vi "LakeShore 370 Curve Manager.vi"(11 "VISA session":refnum<visa-resource-name>) -> ()   [LabVIEW 2020]
doc: "VI to manage calibration curves in Lakeshore model 370 AC resistance Bridge. It will upload, download and display or delete curves. It will always delete a curve before uploading so the input setup may have to be reset after an upload.\nScott Hannahs, <sth@magnet.fsu.edu> NHMFL-FSU, May 2003"
uses:
  Misc Extras/Manufacturer Drivers/LakeShore/Lake Shore Cryotronics 336/Public/Utility/Data Format.ctl
  Sub Controls/ThermListIndex.ctl
  Misc Extras/Manufacturer Drivers/LakeShore/Lake Shore Cryotronics 370/Lake Shore Cryotronics 370.lvlib
panel:
  in  "Done2":bool
  out "XY Graph":cluster{dbl[], dbl[]}(graph)
  out "Curve #":i32[](array[numeric])
  in  "ThermListIndex":T1 max=40 step=20
  in  "stop":bool
  in  "Replace":bool[](array[boolean])=[FALSE, FALSE, FALSE, FALSE, FALSE, FALSE, FALSE, FALSE, FALSE, FALSE, FALSE, FALSE, FALSE, FALSE, FALSE, FALSE, FALSE, FALSE, FALSE, FALSE]
  in  "View":bool[](array[boolean])=[FALSE, FALSE, FALSE, FALSE, FALSE, FALSE, FALSE, FALSE, FALSE, FALSE, FALSE, FALSE, FALSE, FALSE, FALSE, FALSE, FALSE, FALSE, FALSE, FALSE]
  in  "Delete":bool[](array[boolean])=[FALSE, FALSE, FALSE, FALSE, FALSE, FALSE, FALSE, FALSE, FALSE, FALSE, FALSE, FALSE, FALSE, FALSE, FALSE, FALSE, FALSE, FALSE, FALSE, FALSE]
  out "Thermometer List":T3(array[cluster]) {"Temp. Coef" items=["????", "Negative", "Positive"]; "Setpoint Limit" format="%.4f"; "Data Format" items=["mV/K"=1, "V/K"=2, "Ω/K"=3, "Log Ω/K"=4]}
  out "Model":string="LakeShore Model 370"
  out "Info":string="S/N #000000, Software Date: 20030622"
  # "Name"
  # "Serial #"
  # "Data Format"
  # "Setpoint Limit"
  # "Temp. Coef"
  # "`"
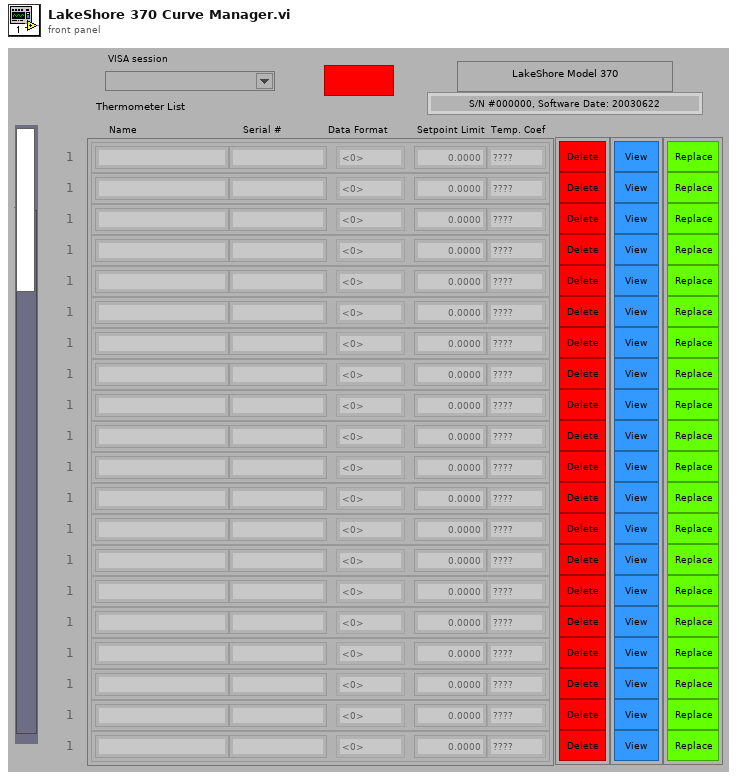
[diagram p1: front panel]
types:
  T1 = typedef "ThermListIndex.ctl" = u32
  T2 = typedef "Data Format.ctl" = u16
  T3 = cluster{"Name":string, "Serial #":string, "Data Format":T2, "Setpoint Limit":dbl, "Temp. Coef":u16}[]
  T4 = cluster{"Curve ID":string, "Serial Number":string, "Data Format":T2, "Setpoint Limit":dbl, "Temp. Coef":u16}[]
  T5 = enum8{"Enabled", "Disabled", "Disabled and Grayed Out"}
  T6 = cluster{"Curve ID":string, "Serial Number":string, "Data Format":T2, "Setpoint Limit":dbl, "Temp. Coef":u16}
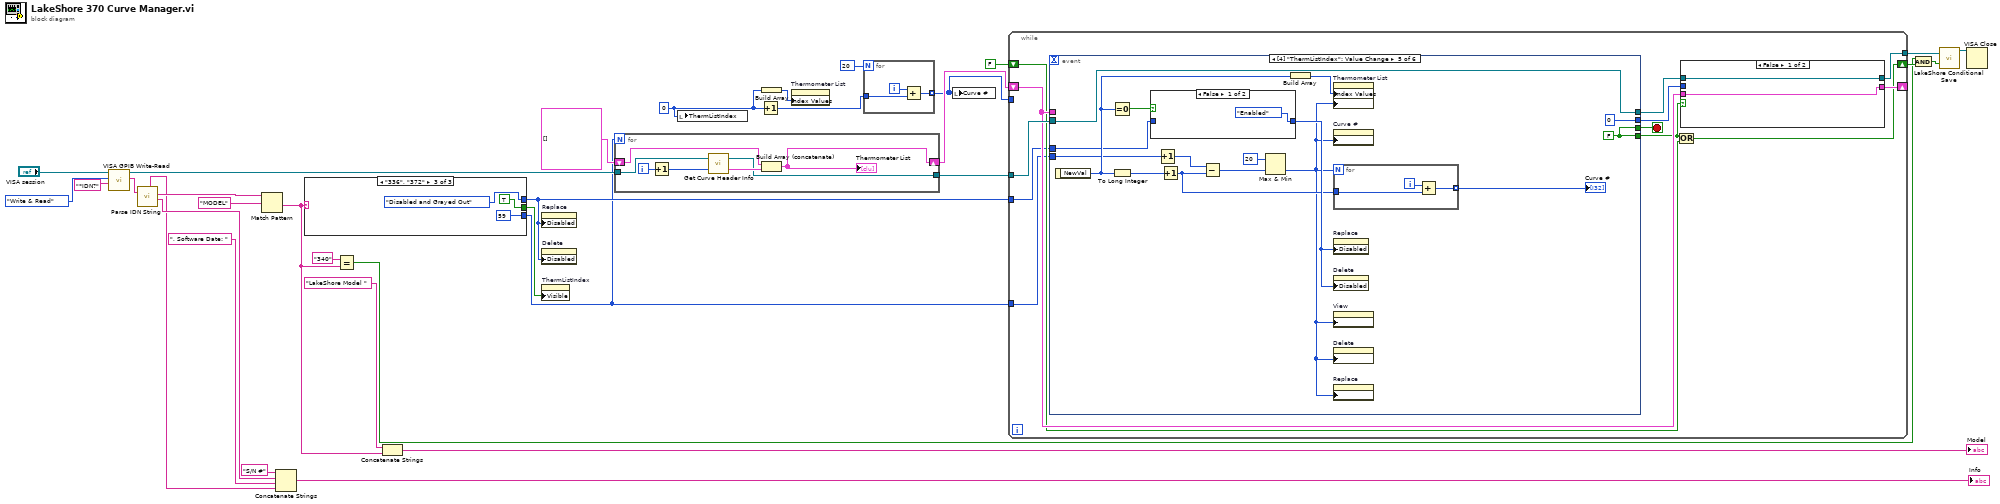
[diagram p0: block diagram]
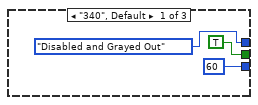
[diagram p2: hidden frame]
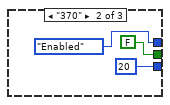
[diagram p3: hidden frame]
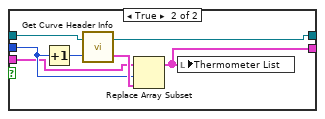
[diagram p4: hidden frame]
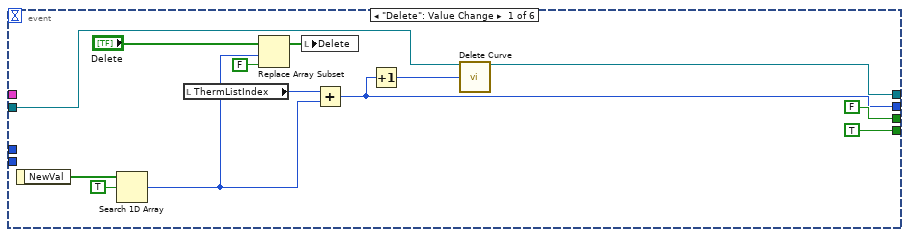
[diagram p5: hidden frame]
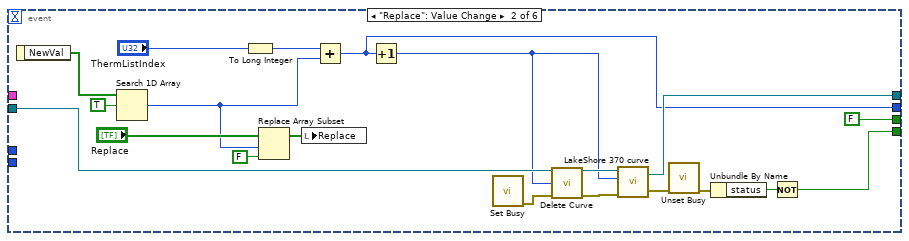
[diagram p6: hidden frame]
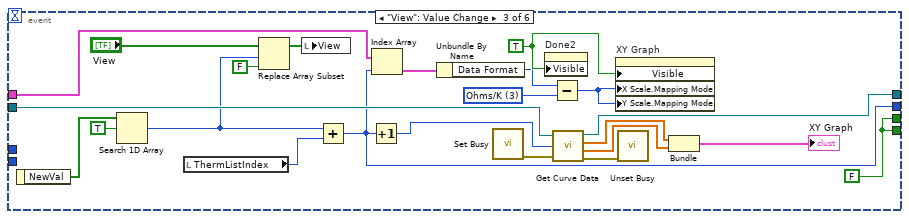
[diagram p7: hidden frame]
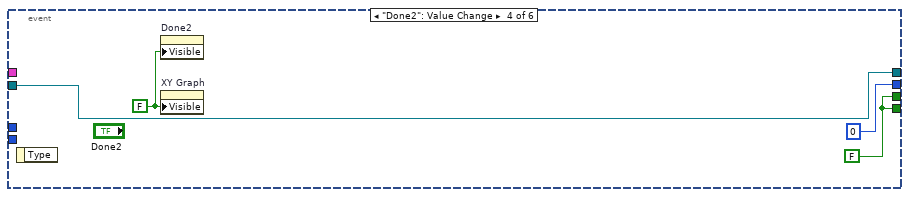
[diagram p8: hidden frame]
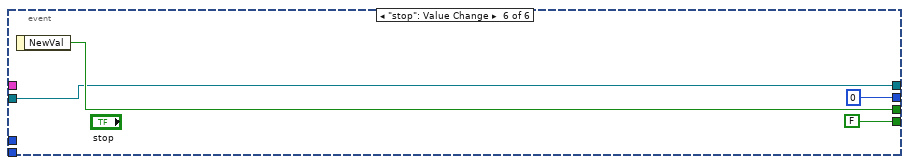
[diagram p10: hidden frame]
diagram:
  w22 = u32 0
  n1 = call "VISA GPIB Write-Read.vi"("Command"="*IDN?" ("String to Write"), "Action"=enum16{"Write", "Read", "Write & Read"}."Write & Read", "VISA resource name"="VISA session") -> ("String Returned"=w10:string, "dup VISA Session"=w27:refnum<visa-resource-name>)  [unwired: 5 in, 2 out]
  n2 = call "Parse IDN String.vi"("IDN String"=w10) -> ("Info"=w7:string, "Model"=w9:string, "Revision"=w6:string)  [unwired: 1 in, 2 out]
  n3 = Match Pattern(string=w9, regular expression="MODEL" ("search string")) -> (after substring=w4:string)  [unwired: 1 in, 3 out]
  n4 = Concatenate Strings("S/N #" ("string"), w7, ", Software Date: " ("string"), w6) -> (→"Info":string)
  n5 = case shown="\"336\", \"372\"" w4 {
    tunnel: [60 20 59] -> w1
    tunnel: [TRUE ("Visible") FALSE ("Visible") TRUE ("Visible")] -> w3
    tunnel: [T5."Disabled and Grayed Out" ("Disabled") T5."Enabled" ("Disabled") T5."Disabled and Grayed Out" ("Disabled")] -> w2
    frame "340", Default {
    }
    frame "370" {
    }
    frame "336", "372" {
    }
  }
  n6 = Equal?(x="340" ("regular expression"), y=w4) -> (x = y?=w13:bool)
  n7 = Concatenate Strings("LakeShore Model " ("string"), w4) -> (→"Model":string)
  n8 = property on="Replace" class="Arr"("Disabled"=w2) -> ()  [unwired: 2 in, 2 out]
  n9 = property on="Delete" class="Arr"("Disabled"=w2) -> ()  [unwired: 2 in, 2 out]
  n10 = property on="ThermListIndex" class="Slide (strict)"("Visible"=w3) -> ()  [unwired: 2 in, 2 out]
  n11 = for {
    N: w1 -> [_]
    tunnel: w27 -> [w49]
    shift-right: [w44] -> w32
    shift-left: T4 [] -> [w43]
    tunnel: [w45] -> w33
    i -> [w48]
    n12 = Increment(x=w48) -> (x+1=w47:i32)
    n13 = call "Get Curve Header Info.vi"("Curve #"=w47, "VISA session"=w49) -> ("Cluster"=w46:T6, "dup VISA session"=w45:refnum<visa-resource-name>)
    n14 = Build Array (concatenate)(w43, w46) -> (w44:T4)
    "Thermometer List" <- w44
  }
  n15 = local write "ThermListIndex"(w22) -> ()
  n16 = Increment(x=w22) -> (x+1=w25:u32)
  n17 = Build Array(w22) -> (w24:u32[])
  n18 = property on="Thermometer List" class="Arr (strict)"("Index Values"=w24) -> ()  [unwired: 2 in, 2 out]
  n19 = for {
    N: 20 -> [_]
    tunnel: w25 -> [w52]
    tunnel: [w50] -> w23 mode=indexing
    i -> [w51]
    n20 = Add(x=w51, y=w52) -> (x+y=w50:u32)
  }
  n21 = local write "Curve #"(w23) -> ()
  n22 = while {
    tunnel: w33 -> [w64]
    shift-right: [w59] -> _
    shift-left: w32 -> [w60]
    tunnel: [w58] -> w18
    tunnel: w23 -> [_]
    shift-right: [w57] -> w20
    shift-left: FALSE ("NewVal") -> [w55]
    tunnel: w2 -> [w54]
    tunnel: w1 -> [w53]
    stop <- w61 stop-if-true
    n23 = event shown="[4] \"ThermListIndex\": Value Change" {
      selector: _ -> [_ _ _ _ _ _]
      dyn-events: _ -> [_ _ _ _ _ _]
      timeout: _ -> [_ _ _ _ _ _]
      tunnel: w64 -> [w84 w90 w127 w130 w149 w156]
      tunnel: [TRUE ("NewVal") w92 w124 w132 w147 FALSE] -> w56
      tunnel: [w74 w97 w109 0 ("index of element") 0 ("index of element") 0 ("index of element")] -> w63
      tunnel: [w83 w104 w126 w130 w149 w156] -> w62
      tunnel: [FALSE ("NewVal") FALSE ("NewVal") w124 w132 w147 w158] -> w61
      tunnel: w60 -> [_ _ w125 _ _ _]
      tunnel: w54 -> [_ _ _ _ w142 _]
      tunnel: w53 -> [_ _ _ _ w138 _]
      event "Delete": Value Change {
        n24 = event-data() -> ("NewVal"=w86:bool[])  [unwired: 1 in]
        n25 = Search 1D Array(1D array=w86, element=TRUE) -> (index of element=w75:i32)  [unwired: 1 in]
        n26 = local read "ThermListIndex"() -> (w76:T1)
        n27 = Replace Array Subset(array="Delete", new element=FALSE ("new element/subarray"), index=w75) -> (w78:bool[])
        n28 = local write "Delete"(w78) -> ()
        n29 = Add(x=w76, y=w75) -> (x+y=w74:T1)
        n30 = Increment(x=w74) -> (x+1=w81:T1)
        n31 = call "Delete Curve.vi"("VISA resource name"=w84, "Curve to Erase (1)"=w81) -> ("VISA resource name out"=w83:refnum<visa-resource-name>)  [unwired: 12 in, 1 out]
      }
      event "Replace": Value Change {
        n32 = event-data() -> ("NewVal"=w105:bool[])  [unwired: 1 in]
        n33 = Search 1D Array(1D array=w105, element=TRUE) -> (index of element=w98:i32)  [unwired: 1 in]
        n34 = To Long Integer(number="ThermListIndex") -> (32bit integer=w96:i32)
        n35 = Replace Array Subset(array="Replace", new element=FALSE ("new element/subarray"), index=w98) -> (w101:bool[])
        n36 = local write "Replace"(w101) -> ()
        n37 = Add(x=w96, y=w98) -> (x+y=w97:i32)
        n38 = Increment(x=w97) -> (x+1=w87:i32)
        n39 = call <vilib>:"Set Busy.vi"() -> ("error out"=w89:errorcluster)  [unwired: 10 in, 1 out]
        n40 = call "Delete Curve.vi"("VISA resource name"=w90, "Curve to Erase (1)"=w87, "error in (no error)"=w89) -> ("VISA resource name out"=w91:refnum<visa-resource-name>, "error out"=w88:errorcluster)  [unwired: 11 in]
        n41 = call "LakeShore 370 curve.vi"("error in (no error)"=w88, "Curve (1)"=w87, "VISA session"=w91) -> ("error out"=w95:errorcluster, "dup VISA session"=w104:refnum<visa-resource-name>)  [unwired: 1 in]
        n42 = call <vilib>:"Unset Busy.vi"("error in (no error)"=w95) -> ("error out"=w94:errorcluster)  [unwired: 10 in]
        n43 = Unbundle By Name(w94) -> ("status"=w93:bool)
        n44 = Not(x=w93) -> (.not. x?=w92:bool)
      }
      event "View": Value Change {
        w116 = T2 3 items=["?????", "????", "???", "Ohms/K", "Log Ohms/K"] ("y")
        w119 = TRUE ("Visible")
        w124 = FALSE ("NewVal")
        n45 = event-data() -> ("NewVal"=w128:bool[])  [unwired: 1 in]
        n46 = Search 1D Array(1D array=w128, element=TRUE) -> (index of element=w110:i32)  [unwired: 1 in]
        n47 = local read "ThermListIndex"() -> (w111:T1)
        n48 = Replace Array Subset(array="View", new element=FALSE ("new element/subarray"), index=w110) -> (w112:bool[])
        n49 = local write "View"(w112) -> ()
        n50 = Add(x=w110, y=w111) -> (x+y=w109:T1)
        n51 = Increment(x=w109) -> (x+1=w123:T1)
        n52 = Index Array(array=w125, index=w109) -> (element=w118:T6)
        n53 = Unbundle By Name(w118) -> ("Data Format"=w117:T2)
        n54 = call <vilib>:"Set Busy.vi"() -> ("error out"=w108:errorcluster)  [unwired: 10 in, 1 out]
        n55 = property on="Done2" class="Bool"("Visible"=w119) -> ()  [unwired: 2 in, 2 out]
        n56 = Subtract(x=w117, y=w116) -> (x-y=w115:T2)
        n57 = call "Get Curve Data.vi"("VISA session"=w127, "Curve #"=w123, "error in (no error)"=w108) -> ("dup VISA session"=w126:refnum<visa-resource-name>, "Temperature"=w121:dbl[], "Resistance"=w122:dbl[], "error out"=w107:errorcluster)
        n58 = property on="XY Graph" class="XYGraph (strict)"("Visible"=w119, "X Scale.Mapping Mode"=w115, "Y Scale.Mapping Mode"=w115) -> ()  [unwired: 2 in, 2 out]
        n59 = call <vilib>:"Unset Busy.vi"("error in (no error)"=w107) -> ()  [unwired: 10 in, 1 out]
        n60 = Bundle("Temperature"=w121, "Resistance"=w122) -> (→"XY Graph":cluster{"Temperature":dbl[], "Resistance":dbl[]})  [unwired: 1 in]
      }
      event "Done2": Value Change {
        w132 = FALSE
        w133 = FALSE ("Visible")
        n61 = event-data() -> ()  [unwired: 1 in, 1 out]
        n62 = property on="Done2" class="Bool"("Visible"=w133) -> ()  [unwired: 2 in, 2 out]
        n63 = property on="XY Graph" class="XYGraph (strict)"("Visible"=w133) -> ()  [unwired: 2 in, 2 out]
      }
      event Value Change {
        w147 = FALSE
        n64 = event-data() -> ("NewVal"=w143:T1)  [unwired: 1 in]
        n65 = Equal To 0?(x=w143) -> (x = 0?=w141:bool)
        n66 = To Long Integer(number=w143) -> (32bit integer=w136:i32)
        n67 = case shown="False" w141 {
          tunnel: w142 -> [_ w151]
          tunnel: [T5."Enabled" ("Disabled") w151] -> w140
          frame False {
          }
          frame True {
          }
        }
        n68 = Increment(x=w138) -> (x+1=w135:i32)
        n69 = Increment(x=w136) -> (x+1=w139:i32)
        n70 = Subtract(x=w135, y=w139) -> (x-y=w137:i32)
        n71 = Max & Min(x=20, y=w137) -> (min(x,y)=w134:i32)  [unwired: 1 out]
        n72 = Build Array(w143) -> (w146:T1[])
        n73 = property on="Thermometer List" class="Arr (strict)"("Index Values"=w146, "Number of Rows"=w134) -> ()  [unwired: 2 in, 2 out]
        n74 = property on="Curve #" class="Arr (strict)"("Number of Rows"=w134) -> ()  [unwired: 2 in, 2 out]
        n75 = for {
          N: w134 -> [_]
          tunnel: w139 -> [w154]
          tunnel: [w152] -> w145 mode=indexing
          i -> [w153]
          n76 = Add(x=w153, y=w154) -> (x+y=w152:i32)
        }
        "Curve #" <- w145
        n77 = property on="Replace" class="Arr"("Disabled"=w140) -> ()  [unwired: 2 in, 2 out]
        n78 = property on="Delete" class="Arr"("Disabled"=w140) -> ()  [unwired: 2 in, 2 out]
        n79 = property on="View" class="Arr"("Number of Rows"=w134) -> ()  [unwired: 2 in, 2 out]
        n80 = property on="Delete" class="Arr"("Number of Rows"=w134) -> ()  [unwired: 2 in, 2 out]
        n81 = property on="Replace" class="Arr"("Number of Rows"=w134) -> ()  [unwired: 2 in, 2 out]
      }
      event "stop": Value Change {
        n82 = event-data() -> ("NewVal"=w158:bool)  [unwired: 1 in]
      }
    }
    n83 = Or(x=w56, y=w55) -> (x .or. y?=w57:bool)
    n84 = case shown="False" w56 {
      tunnel: w63 -> [_ w71]
      tunnel: w62 -> [w65 w70]
      tunnel: w60 -> [w66 w69]
      tunnel: [w66 w67] -> w59
      tunnel: [w65 w68] -> w58
      frame False {
      }
      frame True {
        n85 = Increment(x=w71) -> (x+1=w72:T1)
        n86 = call "Get Curve Header Info.vi"("Curve #"=w72, "VISA session"=w70) -> ("Cluster"=w73:T6, "dup VISA session"=w68:refnum<visa-resource-name>)
        n87 = Replace Array Subset(array=w69, new element=w73, index=w71) -> (w67:T4)
        n88 = local write "Thermometer List"(w67) -> ()
      }
    }
  }
  n89 = And(x=w13, y=w20) -> (x .and. y?=w19:bool)
  n90 = call "LakeShore Conditional Save.vi"("VISA session"=w18, "340? and changed"=w19) -> ("dup VISA session"=w17:refnum<visa-resource-name>)  [unwired: 3 in]
  n91 = VISA Close(VISA resource name=w17) -> ()  [unwired: 1 in, 1 out]
